vi "gfitsio-check-image-for-read.vi"(6 "inc":i32[](array[numeric]), 8 "error in (no error)":errorcluster, 9 "npixels":i32[](array[numeric]), 10 "fpixel":i32[](array[numeric]), 11 "gfits refnum":T1) -> (0 "error out":errorcluster, 1 "lpixel out":i32[](array[numeric]), 2 "fpixel out":i32[](array[numeric]), 3 "dup gfits refnum":T1, 4 "inc out":i32[](array[numeric]), 5 "npixels out":i32[](array[numeric]))   [LabVIEW 2014, in "gfitsio.lvlib"]
doc: "Check the input parameters against the image. If there is a mismatch in dimensionality or if a parameter is out of range for the image return an error. This VI will interpret a -1 for an npixels element to mean the rest of the pixels along that dimension."
uses:
  gfitsio.lvlib
  gfitsio-refnum.ctl
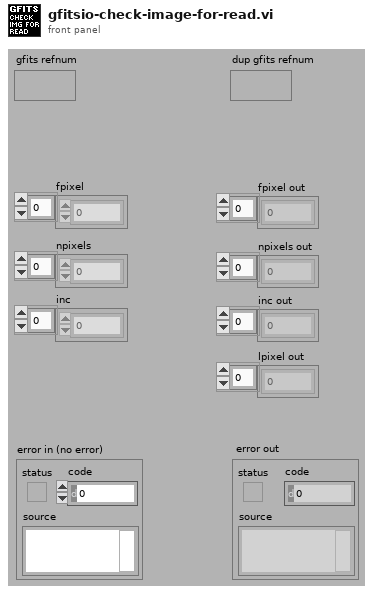
[diagram p1: front panel]
types:
  T1 = typedef "gfitsio.lvlib/gfitsio-refnum.ctl" = refnum<k1>
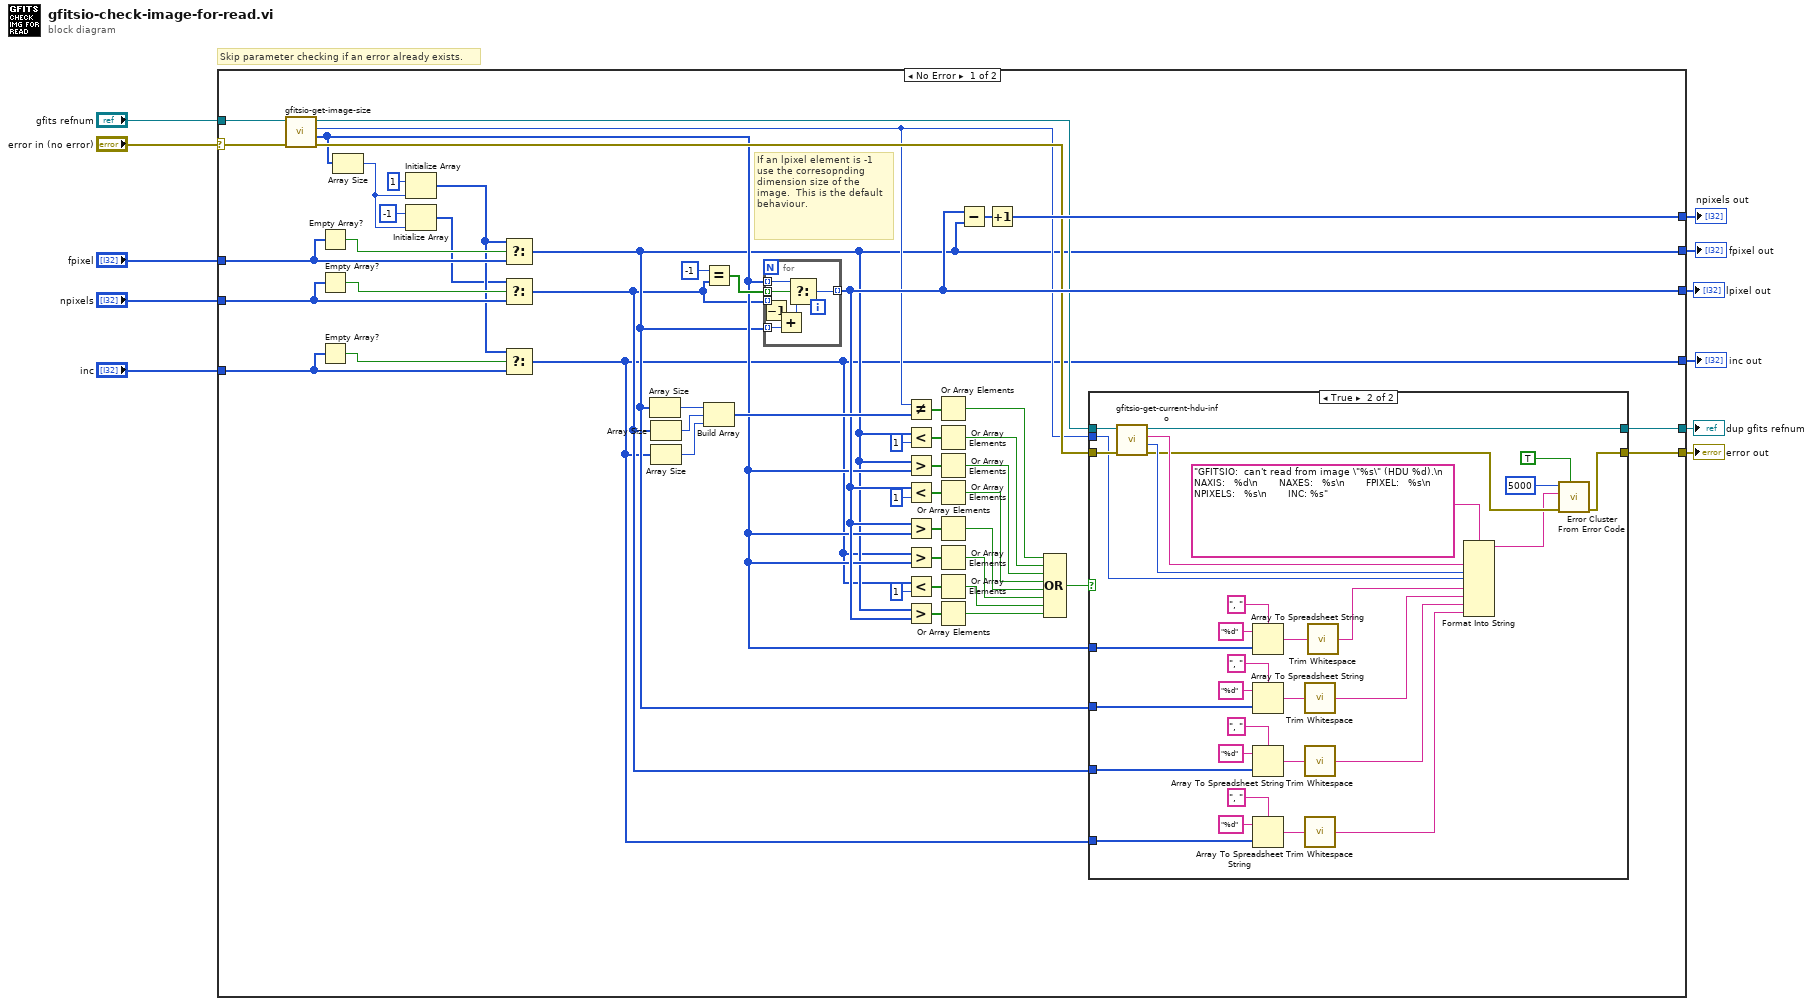
[diagram p0: block diagram]
diagram:
  # "Skip parameter checking if an error already exists."
  n1 = case shown="No Error" "error in (no error)" {
    selector: "error in (no error)" -> [w61 w108]
    tunnel: "gfits refnum" -> [w62 w107]
    tunnel: [w17 w107] -> w6
    tunnel: "fpixel" -> [w37 w106]
    tunnel: "npixels" -> [w36 w104]
    tunnel: "inc" -> [w35 w105]
    tunnel: [w18 w108] -> w11
    tunnel: [w32 _] -> w4
    tunnel: [w12 w105] -> w3
    tunnel: [w14 w106] -> w2
    tunnel: [w30 w104] -> w1
    frame No Error {
      # "If an lpixel element is -1 use the corresopnding dimension size of the image.  This is the default behaviour."
      n2 = call "gfitsio-get-image-size.vi"("error in (no error)"=w61, "gfits refnum"=w62) -> ("error out"=w20:errorcluster, "naxes"=w15:i32[], "naxis"=w16:i32, "dup gfits refnum"=w19:T1)  [unwired: 6 in]
      n3 = Empty Array?(array=w37) -> (empty?=w40:bool)
      n4 = Empty Array?(array=w36) -> (empty?=w39:bool)
      n5 = Empty Array?(array=w35) -> (empty?=w38:bool)
      n6 = Array Size(array=w15) -> (size(s)=w42:i32)
      n7 = Initialize Array(1 ("X"), w42) -> (w34:i32[])
      n8 = Initialize Array(-1 ("element"), w42) -> (w33:i32[])
      n9 = Select(t=w34, s=w40, f=w37) -> (s? t:f=w14:i32[])
      n10 = Select(t=w33, s=w39, f=w36) -> (s? t:f=w13:i32[])
      n11 = Select(t=w34, s=w38, f=w35) -> (s? t:f=w12:i32[])
      n12 = Array Size(array=w14) -> (size(s)=w48:i32)
      n13 = Array Size(array=w13) -> (size(s)=w47:i32)
      n14 = Array Size(array=w12) -> (size(s)=w46:i32)
      n15 = Equal?(x=-1, y=w13) -> (x = y?=w49:bool[])
      n16 = Build Array(w48, w47, w46) -> (w45:i32[])
      n17 = for {
        tunnel: w15 -> [w103] mode=indexing
        tunnel: w49 -> [w102] mode=indexing
        tunnel: w13 -> [w99] mode=indexing
        tunnel: [w101] -> w32 mode=indexing
        tunnel: w14 -> [w100] mode=indexing
        n18 = Decrement(x=w99) -> (x-1=w97:i32)
        n19 = Add(x=w97, y=w100) -> (x+y=w98:i32)
        n20 = Select(t=w103, s=w102, f=w98) -> (s? t:f=w101:i32)
      }
      n21 = Not Equal?(x=w16, y=w45) -> (x != y?=w44:bool[])
      n22 = Less?(x=w14, y=1 ("x")) -> (x < y?=w59:bool[])
      n23 = Greater?(x=w14, y=w15) -> (0:w58:bool[])
      n24 = Less?(x=w32, y=1 ("x")) -> (x < y?=w56:bool[])
      n25 = Greater?(x=w32, y=w15) -> (0:w57:bool[])
      n26 = Greater?(x=w12, y=w15) -> (0:w52:bool[])
      n27 = Less?(x=w12, y=1 ("x")) -> (x < y?=w53:bool[])
      n28 = Greater?(x=w14, y=w32) -> (0:w51:bool[])
      n29 = Or Array Elements(Boolean array=w44) -> (logical OR=w29:bool)
      n30 = Or Array Elements(Boolean array=w59) -> (logical OR=w28:bool)
      n31 = Or Array Elements(Boolean array=w58) -> (logical OR=w27:bool)
      n32 = Or Array Elements(Boolean array=w56) -> (logical OR=w26:bool)
      n33 = Or Array Elements(Boolean array=w57) -> (logical OR=w25:bool)
      n34 = Or Array Elements(Boolean array=w52) -> (logical OR=w24:bool)
      n35 = Or Array Elements(Boolean array=w53) -> (logical OR=w23:bool)
      n36 = Or Array Elements(Boolean array=w51) -> (logical OR=w22:bool)
      n37 = Subtract(x=w32, y=w14) -> (x-y=w31:i32[])
      n38 = Increment(x=w31) -> (x+1=w30:i32[])
      n39 = Compound Arithmetic op=OR(w29, w28, w27, w26, w25, w24, w23, w22) -> (w21:bool)
      n40 = case shown="True" w21 {
        tunnel: w19 -> [w64 w96]
        tunnel: w20 -> [w63 w95]
        tunnel: [w63 w73] -> w18
        tunnel: [w64 w94] -> w17
        tunnel: w16 -> [_ w78]
        tunnel: w15 -> [_ w77]
        tunnel: w14 -> [_ w76]
        tunnel: w13 -> [_ w75]
        tunnel: w12 -> [_ w69]
        frame False {
        }
        frame True {
          n41 = call "gfitsio-get-current-hdu-info.vi"("error in (no error)"=w95, "gfits refnum"=w96) -> ("error out"=w74:errorcluster, "hdu number"=w79:i32, "hdu name"=w80:string, "dup gfits refnum"=w94:T1)  [unwired: 5 in, 1 out]
          n42 = Array To Spreadsheet String(delimiter (Tab)=", ", array=w77, 3:"%d" ("format string")) -> (spreadsheet string=w85:string)
          n43 = Array To Spreadsheet String(delimiter (Tab)=", ", array=w76, 3:"%d" ("format string")) -> (spreadsheet string=w91:string)
          n44 = Array To Spreadsheet String(delimiter (Tab)=", ", array=w75, 3:"%d" ("format string")) -> (spreadsheet string=w84:string)
          n45 = Array To Spreadsheet String(delimiter (Tab)=", ", array=w69, 3:"%d" ("format string")) -> (spreadsheet string=w68:string)
          n46 = call <vilib>:"Trim Whitespace.vi"("string"=w91) -> ("trimmed string"=w82:string)  [unwired: 1 in]
          n47 = call <vilib>:"Trim Whitespace.vi"("string"=w84) -> ("trimmed string"=w83:string)  [unwired: 1 in]
          n48 = call <vilib>:"Trim Whitespace.vi"("string"=w68) -> ("trimmed string"=w65:string)  [unwired: 1 in]
          n49 = call <vilib>:"Trim Whitespace.vi"("string"=w85) -> ("trimmed string"=w81:string)  [unwired: 1 in]
          n50 = Format Into String(format string="GFITSIO:  can't read from image \"%s\" (HDU %d).\n       NAXIS:   %d\n       NAXES:   %s\n       FPIXEL:   %s\n       NPIXELS:   %s\n       INC: %s" ("error message (\"\")"), w80, w79, w78, w81, w82, w83, w65) -> (resulting string=w70:string)  [unwired: 2 in, 1 out]
          n51 = call <vilib>:"Error Cluster From Error Code.vi"("show call chain? (False)"=TRUE, "error in (no error)"=w74, "error message (\"\")"=w70, "error code (0)"=5000) -> ("error out"=w73:errorcluster)  [unwired: 5 in]
        }
      }
    }
    frame Error {
    }
  }
  "error out" <- w11
  "dup gfits refnum" <- w6
  "lpixel out" <- w4
  "inc out" <- w3
  "fpixel out" <- w2
  "npixels out" <- w1
